vi "Set Aircraft RC Override.vi"(8 "Error In":errorcluster, 10 "Auto Override Values":T1, 11 "Aircraft ID":u8) -> (0 "Error Out":errorcluster)   [LabVIEW 2014]
uses:
  Controls/RC Override.ctl
  Controls/Aircraft Mode.ctl
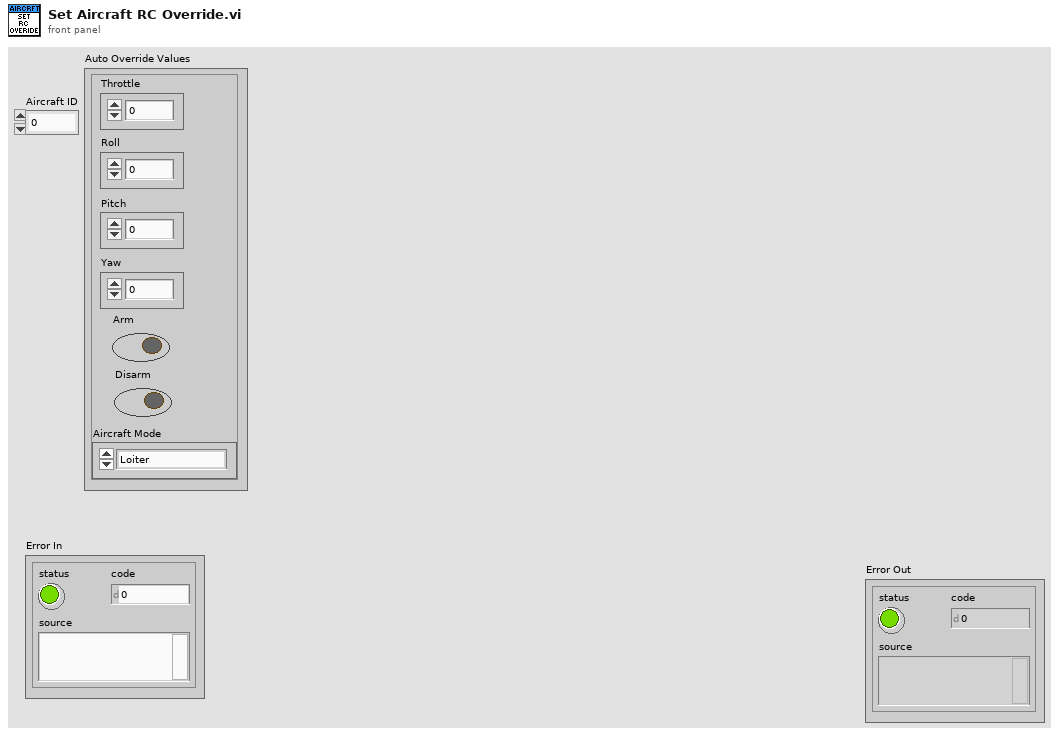
[diagram p1: front panel]
types:
  T1 = typedef "RC Override.ctl" = cluster{"Throttle":u16, "Roll":u16, "Pitch":u16, "Yaw":u16, "Arm":bool, "Disarm":bool, "Aircraft Mode":T2}
  T2 = typedef "Aircraft Mode.ctl" = enum16{"Loiter", "Stabalise", "Failsafe", "Emergency Stop"}
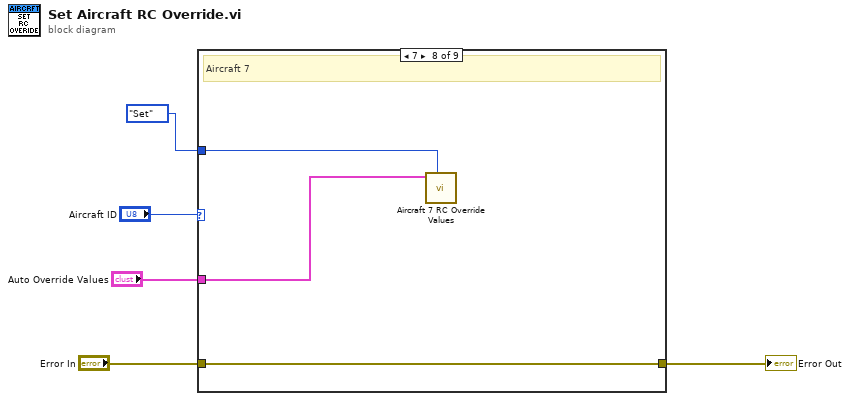
[diagram p0: block diagram]
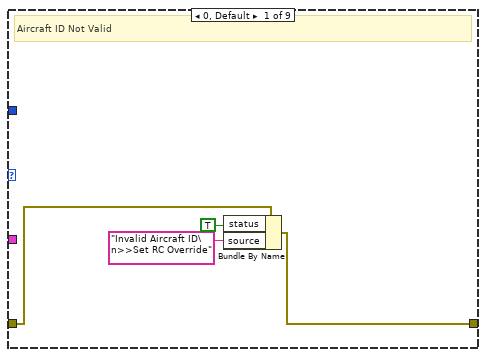
[diagram p2: hidden frame]
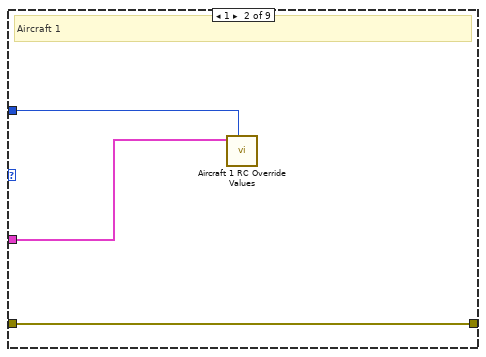
[diagram p3: hidden frame]
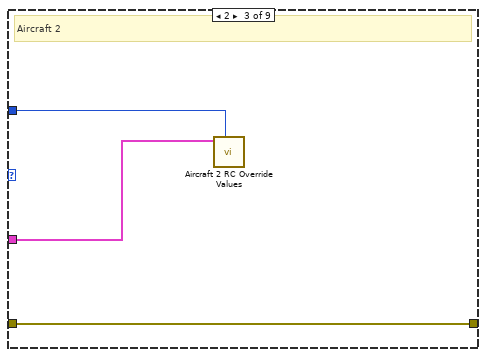
[diagram p4: hidden frame]
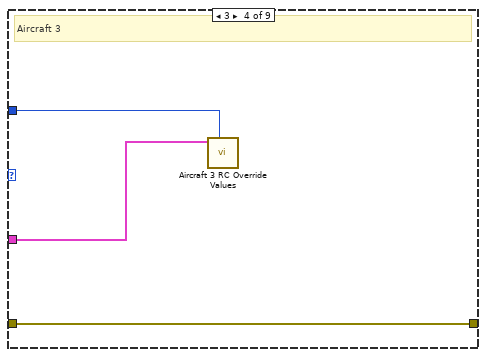
[diagram p5: hidden frame]
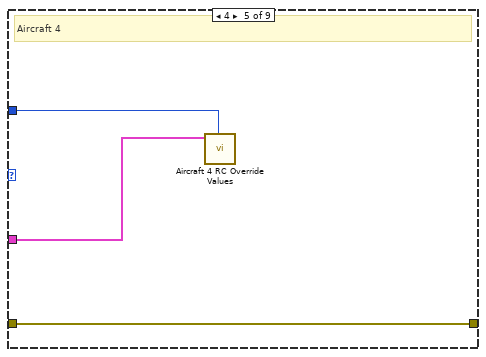
[diagram p6: hidden frame]
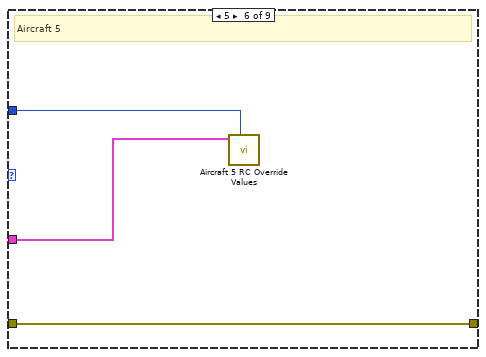
[diagram p7: hidden frame]
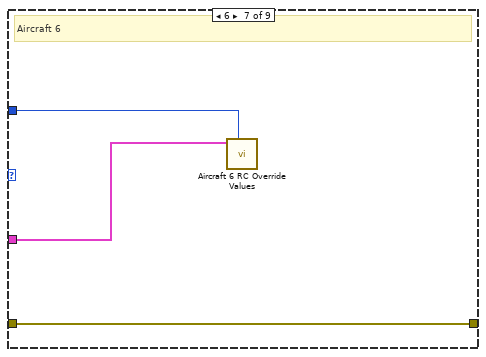
[diagram p8: hidden frame]
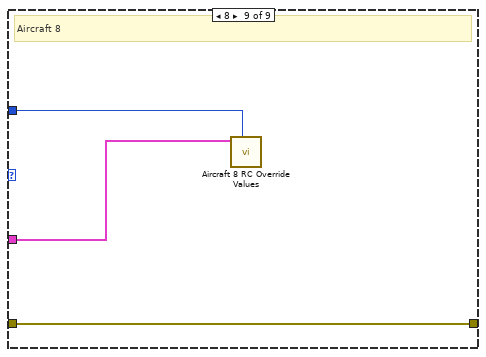
[diagram p9: hidden frame]
diagram:
  n1 = case shown="7" "Aircraft ID" {
    tunnel: [w8 w12 w15 w18 w21 w24 w27 w30 w33] -> w4
    tunnel: "Error In" -> [w9 w12 w15 w18 w21 w24 w27 w30 w33]
    tunnel: enum16{"Get", "Set"}."Set" ("Method") -> [_ w11 w14 w17 w20 w23 w26 w29 w32]
    tunnel: "Auto Override Values" -> [_ w10 w13 w16 w19 w22 w25 w28 w31]
    frame 0, Default {
      # "Aircraft ID Not Valid"
      n2 = Bundle By Name(cluster=w9, "status"=TRUE, "source"="Invalid Aircraft ID\n>>Set RC Override") -> (w8:errorcluster)
    }
    frame 1 {
      # "Aircraft 1"
      n3 = call "Aircraft 1 RC Override Values.vi"("Method"=w11, "Auto Override Values"=w10) -> ()  [unwired: 9 in, 1 out]
    }
    frame 2 {
      # "Aircraft 2"
      n4 = call "Aircraft 2 RC Override Values.vi"("Method"=w14, "Auto Override Values"=w13) -> ()  [unwired: 9 in, 1 out]
    }
    frame 3 {
      # "Aircraft 3"
      n5 = call "Aircraft 3 RC Override Values.vi"("Method"=w17, "Auto Override Values"=w16) -> ()  [unwired: 9 in, 1 out]
    }
    frame 4 {
      # "Aircraft 4"
      n6 = call "Aircraft 4 RC Override Values.vi"("Method"=w20, "Auto Override Values"=w19) -> ()  [unwired: 9 in, 1 out]
    }
    frame 5 {
      # "Aircraft 5"
      n7 = call "Aircraft 5 RC Override Values.vi"("Method"=w23, "Auto Override Values"=w22) -> ()  [unwired: 9 in, 1 out]
    }
    frame 6 {
      # "Aircraft 6"
      n8 = call "Aircraft 6 RC Override Values.vi"("Method"=w26, "Auto Override Values"=w25) -> ()  [unwired: 9 in, 1 out]
    }
    frame 7 {
      # "Aircraft 7"
      n9 = call "Aircraft 7 RC Override Values.vi"("Method"=w29, "Auto Override Values"=w28) -> ()  [unwired: 9 in, 1 out]
    }
    frame 8 {
      # "Aircraft 8"
      n10 = call "Aircraft 8 RC Override Values.vi"("Method"=w32, "Auto Override Values"=w31) -> ()  [unwired: 9 in, 1 out]
    }
  }
  "Error Out" <- w4
